vi "To Table Test.vi"() -> ()   [LabVIEW 2015, in "User Control Module Test.lvlib"]
uses:
  User Control Module Test.lvlib
  Program Files (x86)/National Instruments/LabVIEW 2015/ProjectTemplates/Source/dcaf configurable plugin module/IO Plugin/editor node/tag bus configurable plugin editor node.lvclass
  <vilib>/NI/Module Execution Interface/Engine Configuration/engine configuration.lvclass
  <vilib>/NI/Tag Bus/tag/tag descriptor.lvclass
  <vilib>/NI/Configuration Framework/serializable configuration/NISE_CEF_serializable configuration.lvclass
panel:
  out "error out":errorcluster
  out "table":string[][](array[string])
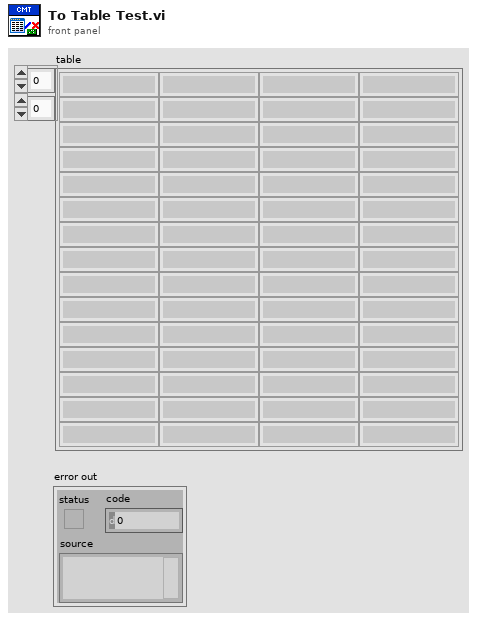
[diagram p1: front panel]
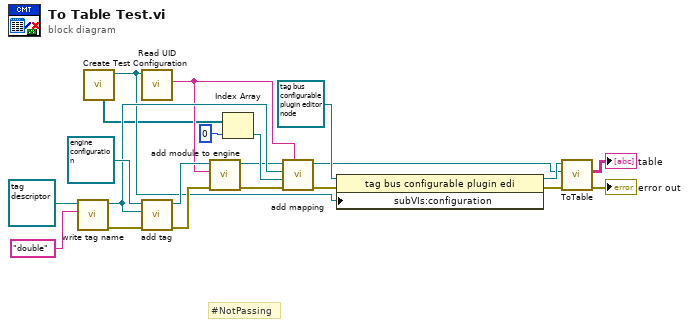
[diagram p0: block diagram]
diagram:
  # "#NotPassing"
  n1 = call <vilib>:"write tag name.vi"("name"="double", "system tag in"=refnum<class "tag descriptor.lvclass"> refnum ("tag descriptor")) -> ("error out"=w5:errorcluster, "system tag out"=w12:refnum<class "tag descriptor.lvclass">)  [unwired: 8 in]
  n2 = call "Create Test Configuration.vi"() -> ("Module"=w4:refnum<class "user control module configuration.lvclass">, "Channels"=w3:refnum<class "TBM channel.lvclass">[])  [unwired: 6 in, 4 out]
  n3 = call <vilib>:"Read UID.vi"("configuration in"=w4) -> ("instance id"=w8:string)  [unwired: 8 in, 2 out]
  n4 = call <vilib>:"add tag.vi"("error in"=w5, "tag descriptor"=w12, "engine configuration in"=refnum<class "engine configuration.lvclass"> refnum ("engine configuration")) -> ("error out"=w6:errorcluster, "engine configuration out"=w10:refnum<class "engine configuration.lvclass">)  [unwired: 7 in]
  n5 = call-dynamic "add module to engine.vi"("error in"=w6, "module ID"=w8, "engine configuration in"=w10) -> ("error out"=w7:errorcluster, "engine configuration out"=w9:refnum<class "engine configuration.lvclass">)  [unwired: 7 in]
  n6 = Index Array(array=w3, index=0) -> (element=w13:refnum<class "TBM channel.lvclass">)
  n7 = call <vilib>:"add mapping.vi"("owner ID"=w8, "error in"=w7, "channel"=w13, "tag descriptor"=w12, "engine configuration"=w9) -> ("error out"=w1:errorcluster, "engine configuration out"=w11:refnum<class "engine configuration.lvclass">)  [unwired: 5 in]
  n8 = property class="tag bus configurable plugin edi"(reference=refnum<class "tag bus configurable plugin editor node.lvclass"> refnum ("node in"), error in=w1, "subVIs:configuration"=w4) -> (reference out=w20:refnum<class "tag bus configurable plugin editor node.lvclass">, error out=w2:errorcluster)
  n9 = call-dynamic "ToTable.vi"("error in"=w2, "variant"=w11, "node in"=w20) -> ("error out"=→"error out":errorcluster, "table"=→"table":string[][])  [unwired: 6 in, 1 out]
